vi "Create.vi"(8 "error in (no error)":errorcluster) -> (0 "error out":errorcluster, 3 "CameraManager":refnum<data-value>)   [LabVIEW 2020, in "g_ar_toolkit.capture.lvlib" / "CameraManager.lvclass"]
doc: "Create Camera Manager instance"
uses:
  CameraManager.lvclass
  CameraManager.lvclass/CameraManager.ctl
  bin/g_ar_toolkit.1.32.dll
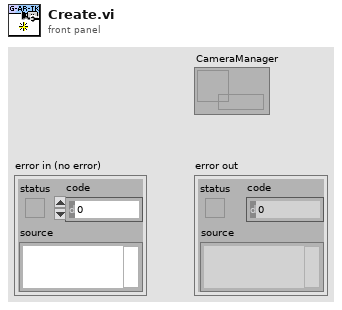
[diagram p1: front panel]
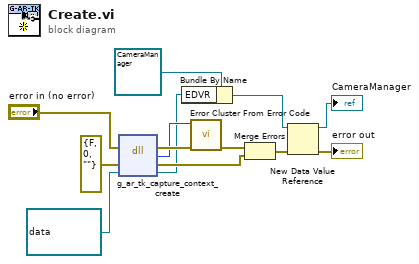
[diagram p0: block diagram]
diagram:
  n1 = dll-call lib="C:/serenial/libraries/g-augmented-reality-toolkit/LabVIEW/bin/g_ar_toolkit.1.*.*" fn="g_ar_tk_capture_context_create"(error in="error in (no error)", "error_cluster"=errorcluster {"status"=FALSE, "code"=0, "source"=""} ("error constant"), "EDVR"=refnum<data-value> refnum) -> (error out=w10:errorcluster, "MgErr"=w9:i32, "error_cluster"=w6:errorcluster, "EDVR"=w2:refnum<data-value>)  [unwired: 2 in, 1 out]
  n2 = Bundle By Name(cluster=refnum<class "CameraManager.lvclass"> refnum ("CameraManager out"), "EDVR"=w2) -> (w5:refnum<class "CameraManager.lvclass">)
  n3 = call <vilib>:"Error Cluster From Error Code.vi"("error in (no error)"=w10, "error code (0)"=w9) -> ("error out"=w8:errorcluster)  [unwired: 7 in]
  n4 = Merge Errors(w8, w6) -> (w3:errorcluster)
  n5 = New Data Value Reference(data value=w5, error in=w3) -> (data value reference=→"CameraManager":refnum<data-value>, error out=→"error out":errorcluster)
